vi "hello_world.vi"() -> ()   [LabVIEW 2021]
panel:
  out "String":string
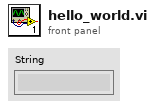
[diagram p1: front panel]
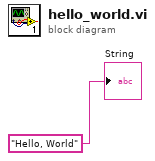
[diagram p0: block diagram]
diagram:
  "String" <- "Hello, World"
